vi "Check_EnFlo_Arm.vi"() -> ()   [LabVIEW 2014]
uses:
  Gen Trav/Trav_mode.ctl
  Controls/Home.ctl
  Gen Trav/Route mapping/Route_mapping_global.vi
  Globals/Trav_pos_global.vi
  ADAM Serial/Instrument drivers/Traverses/~subVIs/DriveConfigGlobal.vi
panel:
  out "Position Output XYZ":dbl[](array[numeric]) format="%.2f"
  in  "Mode":T1(ring)
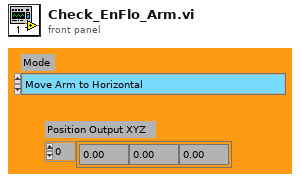
[diagram p1: front panel]
types:
  T1 = enum16{"Move Arm to Horizontal", "Teach Traverse That Arm is Level"}
  T2 = typedef "Tunnel_Coordinates.ctl" = enum16{"Work in Tunnel Coordinates", "Work in Model Coordinates"}
  T3 = typedef "Box_size.ctl" = cluster{"Max":dbl, "Min":dbl}[]
  T4 = typedef "Exclude_cluster.ctl" = cluster{"Sizes":T3, "Name":string, "Exclude Type":T5}
  T5 = typedef "Exclusion_type.ctl" = enum16{"Exclude completely", "Allow only vertical moves"}
  T6 = typedef "Trav_mode.ctl" = enum16{"Move traverse", "Read traverse position", "Teach Position"}
  T7 = enum16{"Load setup from excel file", "Save setup to excel file"}
  T8 = typedef "Home.ctl" = enum16{"Don't Home", "Home  +X", "Home  -X", "Home  +Y", "Home  -Y", "Home  +Z", "Home  -Z"}
  T9 = typedef "AxisConfigCluster.ctl" = cluster{"Channel Properties":T10, "Static Drive Configuration":T11}
  T10 = typedef "DriveProperties.ctl" = cluster{"Channel Name":string, "Vel. Default":dbl, "Acc. Default":dbl, "Vel. Max":dbl, "Vel. Min":dbl, "Acc. Max":dbl, "Acc. Min":dbl, "Pulses/unit":dbl, "Address":u8, "Pulse Offset":i32, "Pos Tolerance":dbl, "Pulses/rev":dbl, "Backlash/Eng units":dbl, "Current Pos":dbl, "Ch Status":enum16{"Active", "Offline", "Simulate"}, "Port Name":string, "Axis Transform mode":string, "Metadata Ch Name":string, "Type":string}
  T11 = typedef "DriveStaticConfig.ctl" = cluster{"Correction Gain % (CG)":u16, "Dead Band (DB)":i32, "Dead Band Window (DW)":i32, "Encoder Resolution (ER)":i32, "Step Mode  (FSB)":u16, "Position Maintenance (FSC)":u16, "Stop on Stall (FSD)":u16, "Activate OP1 on stall (FSE)":u16, "Stop on Trigger 3 (FSF)":u16, "OP2 in Deadband (FSG)":u16, "Stall Detect (FSH)":u16, "Limit Disable (LD)":u16, "Motor Resolution (MR)":enum16{"200", "400", "1000", "2000", "4000", "5000", "10000", "12800", "18000", "20000", "21600", "25000", "25400", "25600", "36000", "50000", "278528", "425984", "507904", "614400", "655360", "819200", "1024000"}, "Limit Switch Sense (OSA)":u16, "Home Position (OSB)":u16, "Home Switch Sense (OSC)":u16, "Encoder Z for Home (OSD)":u16, "Reference edge of Home (OSH)":u16, "RS232 Echo Control (SSA)":u16, "Buffer at Limit (SSG)":u16, "Buffer at Stop (SSH)":u16, "Indexer Mode  (FSA)":u16, "Type":string, "ConfigString":string, "De Power Motor":enum16{"TRUE", "FALSE"}}
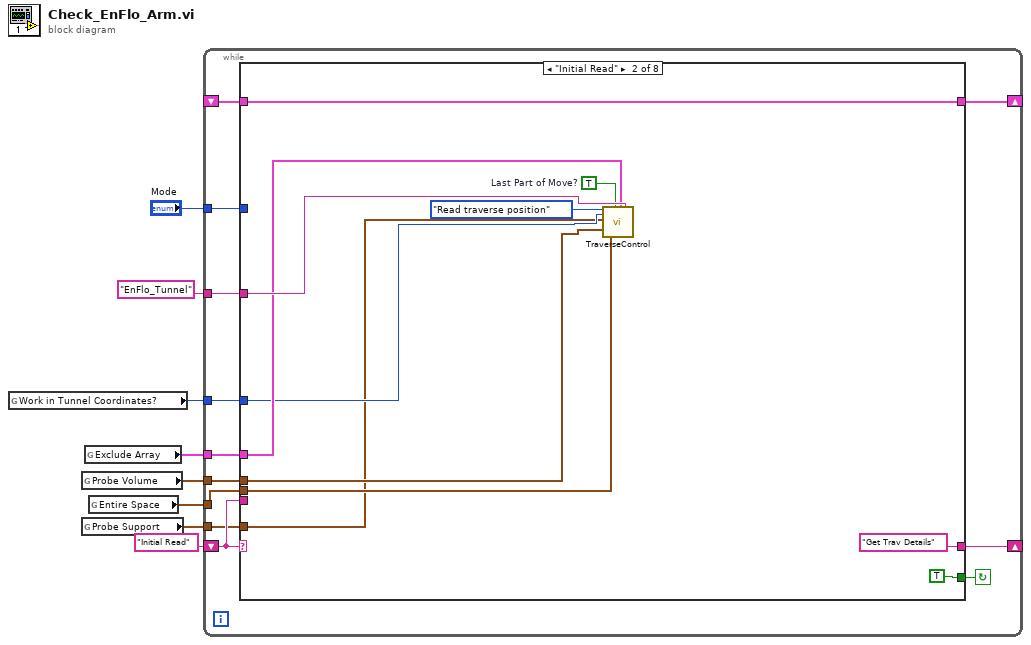
[diagram p0: block diagram]
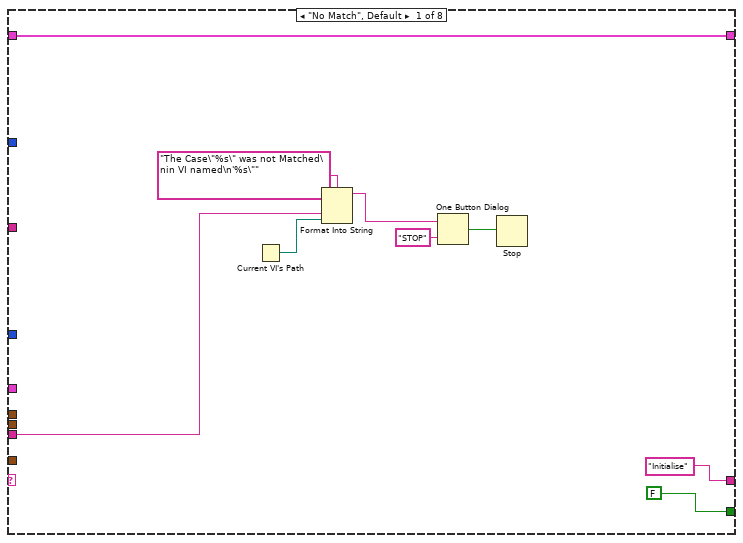
[diagram p2: hidden frame]
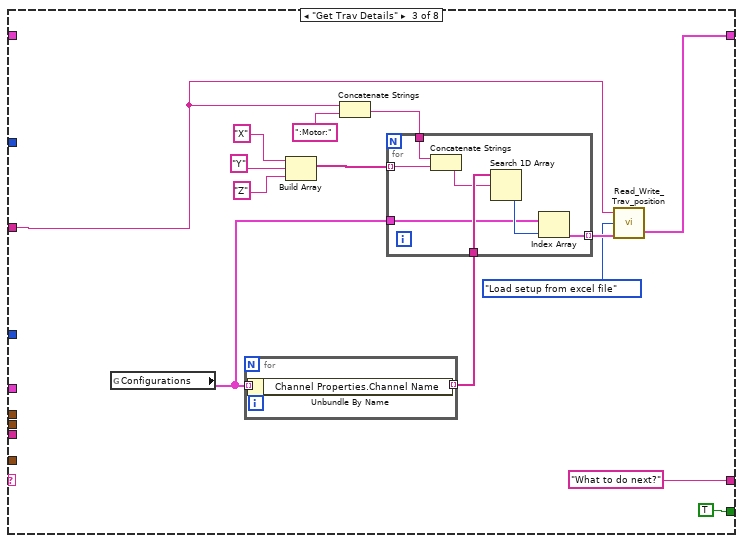
[diagram p3: hidden frame]
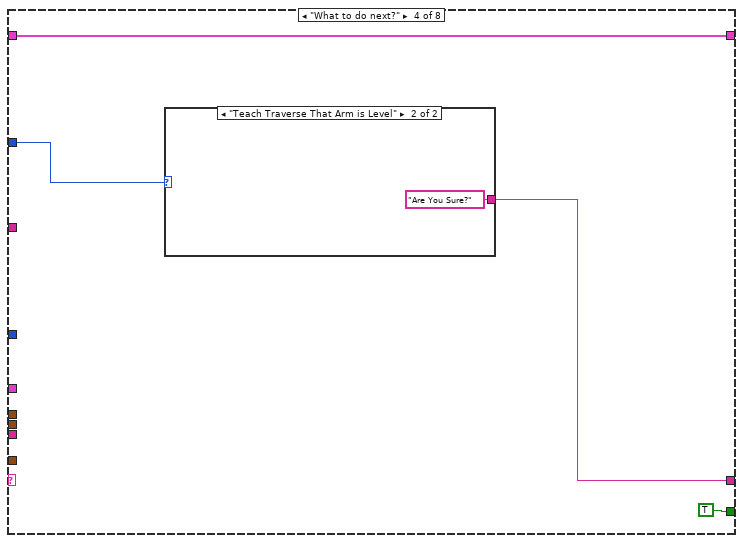
[diagram p4: hidden frame]
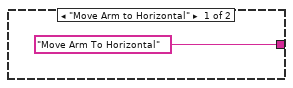
[diagram p5: hidden frame]
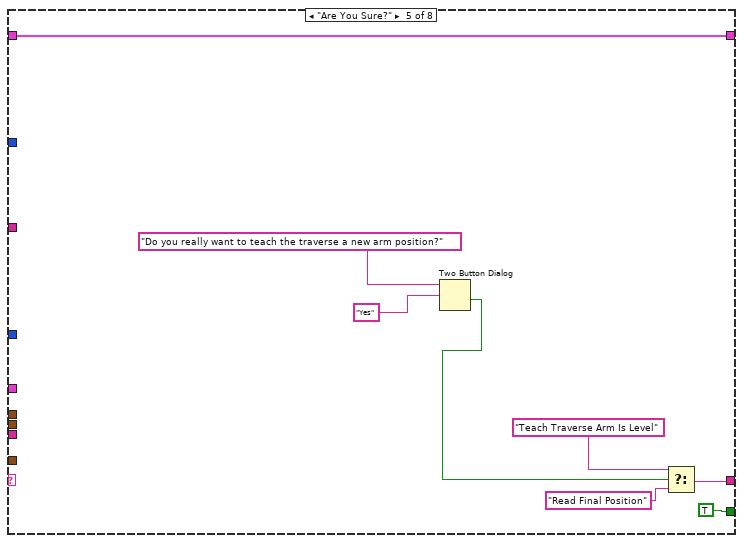
[diagram p6: hidden frame]
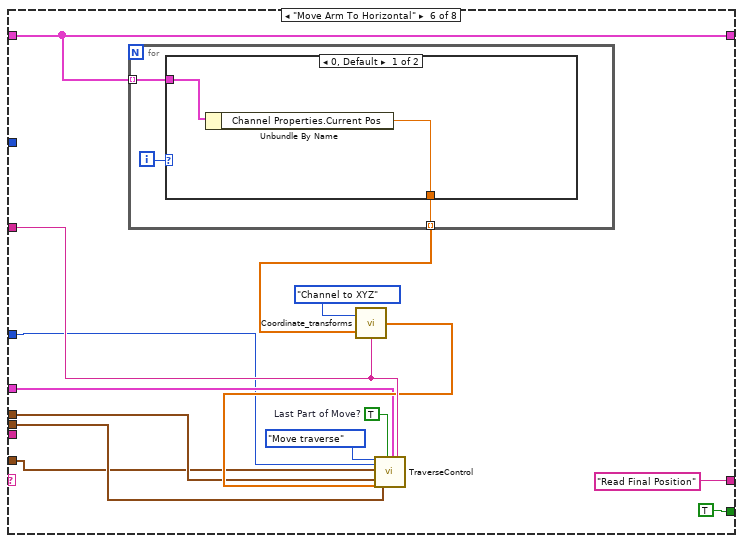
[diagram p7: hidden frame]
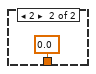
[diagram p8: hidden frame]
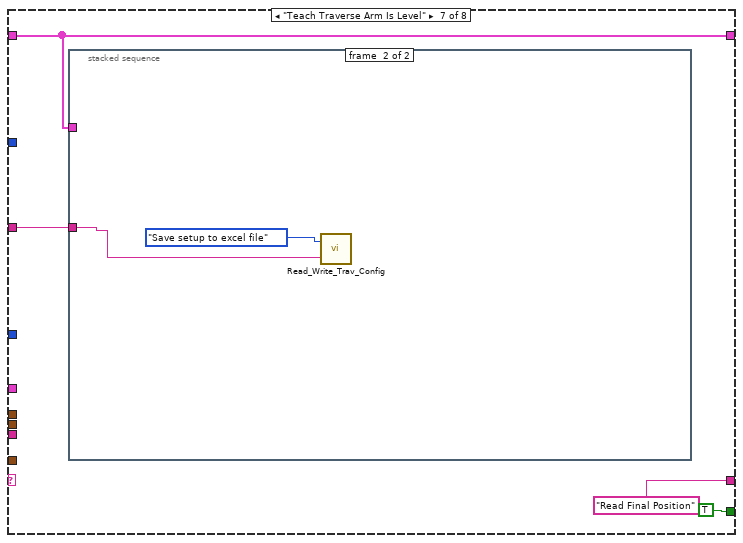
[diagram p9: hidden frame]
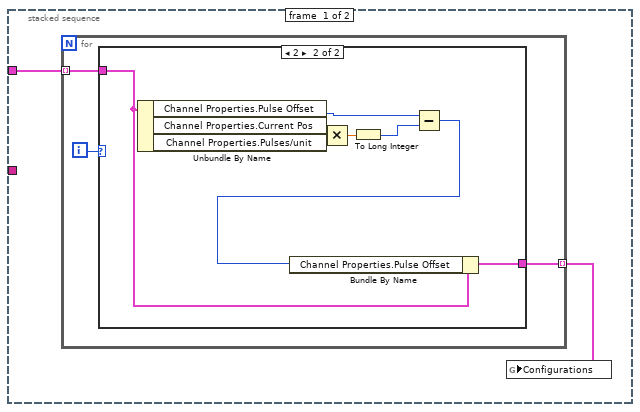
[diagram p10: hidden frame]
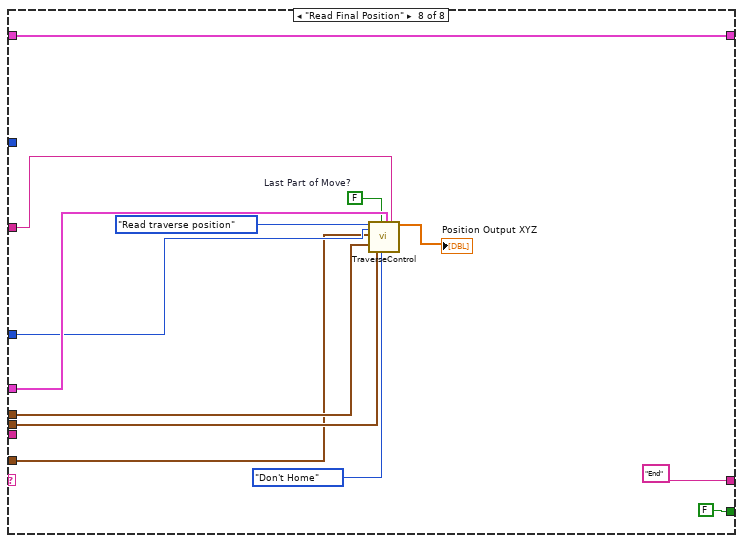
[diagram p12: hidden frame]
diagram:
  n1 = global read "Trav_pos_global.vi" "Work in Tunnel Coordinates?"() -> (w2:T2)
  n2 = global read "Route_mapping_global.vi" "Probe Volume"() -> (w4:T3)
  n3 = global read "Route_mapping_global.vi" "Probe Support"() -> (w1:T3)
  n4 = global read "Route_mapping_global.vi" "Exclude Array"() -> (w5:T4[])
  n5 = global read "Route_mapping_global.vi" "Entire Space"() -> (w3:T3)
  n6 = while {
    tunnel: "Mode" -> [w14]
    shift-left: _ -> [w15]
    shift-right: [w16] -> _
    tunnel: "EnFlo_Tunnel" ("Traverse Name") -> [w17]
    shift-left: "Initial Read" -> [w18]
    shift-right: [w19] -> _
    tunnel: w5 -> [w13]
    tunnel: w4 -> [w12]
    tunnel: w3 -> [w11]
    tunnel: w2 -> [w10]
    tunnel: w1 -> [w9]
    stop <- w20 continue-if-true
    n7 = case shown="\"Initial Read\"" w18 {
      tunnel: [FALSE TRUE TRUE TRUE TRUE TRUE TRUE FALSE] -> w20
      tunnel: ["Initialise" "Get Trav Details" "What to do next?" w65 w71 "Read Final Position" "Read Final Position" "End"] -> w19
      tunnel: w18 -> [w24 _ _ _ _ _ _ _]
      tunnel: w17 -> [_ w36 w42 _ _ w86 w98 w127]
      tunnel: [w21 w37 w41 w64 w76 w89 w99 w126] -> w16
      tunnel: w15 -> [w21 w37 _ w64 w76 w89 w99 w126]
      tunnel: w14 -> [_ _ _ w66 _ _ _ _]
      tunnel: w13 -> [_ w35 _ _ _ w83 _ w124]
      tunnel: w12 -> [_ w33 _ _ _ w82 _ w122]
      tunnel: w11 -> [_ w34 _ _ _ w81 _ w123]
      tunnel: w10 -> [_ w32 _ _ _ w80 _ w121]
      tunnel: w9 -> [_ w31 _ _ _ w79 _ w120]
      frame "No Match", Default {
        n8 = Current VI's Path() -> (path=w23:path)
        n9 = Format Into String(format string="The Case\"%s\" was not Matched\nin VI named\n'%s\"" ("Format String"), w24, w23) -> (resulting string=w27:string)  [unwired: 2 in, 1 out]
        n10 = One Button Dialog(message=w27, button name ("OK")="STOP") -> (true=w25:bool)
        n11 = Stop(stop? (T)=w25) -> ()
      }
      frame "Initial Read" {
        w30 = TRUE  # Last Part of Move?
        n12 = call "TraverseControl.vi"("Mode"=Trav_mode."Read traverse position", "Work in Tunnel Coordinates?"=w32, "Probe Support"=w31, "Probe Volume"=w33, "Entire Space"=w34, "Last Part of Move?"=w30, "Exclude Array"=w35, "Traverse Name"=w36) -> ()  [unwired: 10 in, 2 out]
      }
      frame "Get Trav Details" {
        n13 = global read "DriveConfigGlobal.vi" "Configurations"() -> (w45:T9[])
        n14 = for {
          tunnel: w45 -> [w56] mode=indexing
          tunnel: [w55] -> w46 mode=indexing
          n15 = Unbundle By Name(w56) -> ("Channel Properties.Channel Name"=w55:string)
        }
        n16 = Build Array("X", "Y", "Z") -> (w51:string[])
        n17 = Concatenate Strings(w42, ":Motor:") -> (w50:string)
        n18 = for {
          tunnel: w51 -> [w63] mode=indexing
          tunnel: w50 -> [w62]
          tunnel: w46 -> [w61]
          tunnel: w45 -> [w58]
          tunnel: [w57] -> w44 mode=indexing
          n19 = Concatenate Strings(w62, w63) -> (w60:string)
          n20 = Search 1D Array(1D array=w61, element=w60) -> (index of element=w59:i32)  [unwired: 1 in]
          n21 = Index Array(array=w58, index=w59) -> (element=w57:T9)
        }
        n22 = call "Read_Write_Trav_position.vi"("Matched Configurations In"=w44, "Mode"=T7."Load setup from excel file", "Traverse Name"=w42) -> ("Matched Configurations Out"=w41:T9[])  [unwired: 1 in]
      }
      frame "What to do next?" {
        n23 = case shown="\"Teach Traverse That Arm is Level\"" w66 {
          tunnel: ["Move Arm To Horizontal" "Are You Sure?"] -> w65
          frame "Move Arm to Horizontal" {
          }
          frame "Teach Traverse That Arm is Level" {
          }
        }
      }
      frame "Are You Sure?" {
        n24 = Two Button Dialog(message="Do you really want to teach the traverse a new arm position?", 2:"Yes" ("T button name (\"OK\")")) -> (T button?=w73:bool)  [unwired: 1 in]
        n25 = Select(t="Teach Traverse Arm Is Level", s=w73, f="Read Final Position") -> (s? t:f=w71:string)
      }
      frame "Move Arm To Horizontal" {
        w78 = TRUE  # Last Part of Move?
        n26 = for {
          tunnel: w89 -> [w93] mode=indexing
          tunnel: [w92] -> w87 mode=indexing
          i -> [w94]
          n27 = case shown="0, Default" w94 {
            tunnel: w93 -> [w96 _]
            tunnel: [w95 0.0 ("Current Pos")] -> w92
            frame 0, Default {
              n28 = Unbundle By Name(w96) -> ("Channel Properties.Current Pos"=w95:dbl)
            }
            frame 2 {
            }
          }
        }
        n29 = call "Coordinate_transforms.vi"("Traverse Name"=w86, "Input"=w87, "Mode"=enum16{"XYZ to Channel", "Channel to XYZ"}."Channel to XYZ") -> ("Output"=w85:dbl[])
        n30 = call "TraverseControl.vi"("Mode"=Trav_mode."Move traverse", "Work in Tunnel Coordinates?"=w80, "Probe Support"=w79, "Probe Volume"=w82, "Position input XYZ"=w85, "Entire Space"=w81, "Last Part of Move?"=w78, "Exclude Array"=w83, "Traverse Name"=w86) -> ()  [unwired: 9 in, 2 out]
      }
      frame "Teach Traverse Arm Is Level" {
        n31 = stacked-sequence {
          tunnel: w99 -> [w103 _]
          tunnel: w98 -> [_ w116]
          frame #0 {
            n32 = for {
              tunnel: w103 -> [w105] mode=indexing
              tunnel: [w104] -> w102 mode=indexing
              i -> [w106]
              n33 = case shown="2" w106 {
                tunnel: w105 -> [w107 w112]
                tunnel: [w107 w108] -> w104
                frame 0, Default {
                }
                frame 2 {
                  n34 = Unbundle By Name(w112) -> ("Channel Properties.Pulse Offset"=w113:i32, "Channel Properties.Current Pos"=w115:dbl, "Channel Properties.Pulses/unit"=w114:dbl)
                  n35 = Multiply(x=w115, y=w114) -> (x*y=w111:dbl)
                  n36 = To Long Integer(number=w111) -> (32bit integer=w110:i32)
                  n37 = Subtract(x=w113, y=w110) -> (x-y=w109:i32)
                  n38 = Bundle By Name(cluster=w112, "Channel Properties.Pulse Offset"=w109) -> (w108:T9)
                }
              }
            }
            n39 = global write "DriveConfigGlobal.vi" "Configurations"(w102) -> ()
          }
          frame #1 {
            n40 = call "Read_Write_Trav_Config.vi"("Traverse Name"=w116, "Mode"=T7."Save setup to excel file") -> ()  [unwired: 1 in]
          }
        }
      }
      frame "Read Final Position" {
        w118 = FALSE  # Last Part of Move?
        n41 = call "TraverseControl.vi"("Mode"=Trav_mode."Read traverse position", "Work in Tunnel Coordinates?"=w121, "Probe Support"=w120, "Probe Volume"=w122, "Entire Space"=w123, "Last Part of Move?"=w118, "Home"=Home."Don't Home", "Exclude Array"=w124, "Traverse Name"=w127) -> ("Position Output XYZ"=→"Position Output XYZ":dbl[])  [unwired: 9 in, 1 out]
      }
    }
  }
